vi "Get_Result_Bool.vi"(8 "error in (no error)":errorcluster caption="错误输入（无错误）", 10 "结果数组":bool[][](array[boolean])) -> (0 "error out":errorcluster caption="错误输出", 2 "数组":bool[](array[boolean]))   [LabVIEW 2018]
panel:
  in  "添加的数组":bool[][](array[boolean])
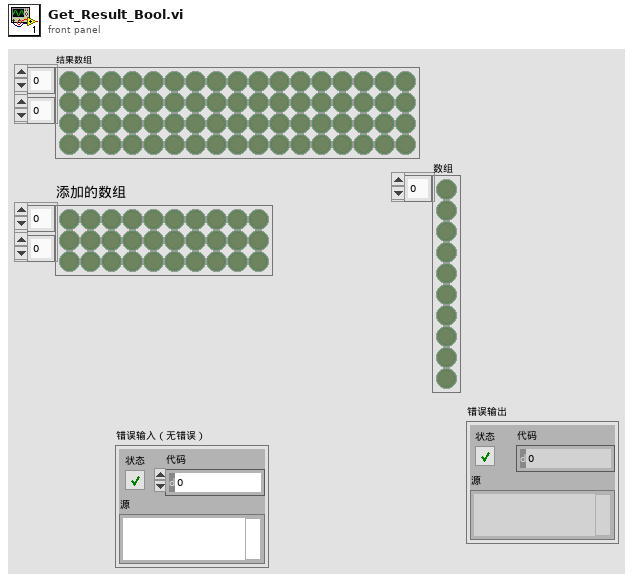
[diagram p1: front panel]
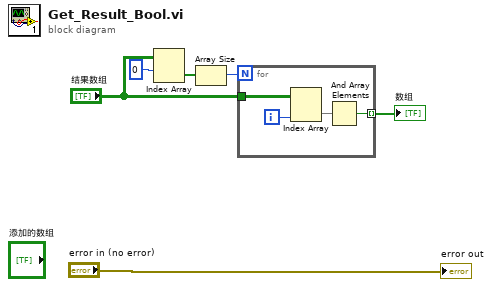
[diagram p0: block diagram]
diagram:
  n1 = Index Array(array="结果数组", index (row)=0 ("索引 (行)")) -> (element=w5:bool[])  [unwired: 1 in]
  n2 = Array Size(array=w5) -> (size(s)=w4:i32)
  n3 = for {
    N: w4 -> [_]
    tunnel: "结果数组" -> [w10]
    tunnel: [w7] -> w2 mode=indexing
    i -> [w9]
    n4 = Index Array(array=w10, index (col)=w9) -> (element=w8:bool[])  [unwired: 1 in]
    n5 = And Array Elements(Boolean array=w8) -> (logical AND=w7:bool)
  }
  "数组" <- w2
  "error out" <- "error in (no error)"
